vi "SetValue.vi"(8 "error in":errorcluster, 10 "Value":timestamp, 11 "DateTimeMeasure in":refnum<class "DateTimeMeasure.lvclass">) -> (0 "error out":errorcluster, 3 "DateTimeMeasure out":refnum<class "DateTimeMeasure.lvclass">)   [LabVIEW 2021, in "ProligentXMLGenerator.lvlib" / "DateTimeMeasure.lvclass"]
doc: "Defines the value acquired by the measure."
uses:
  DateTimeMeasure.lvclass
  DateTimeMeasure.lvclass/DateTimeMeasure.ctl
  Base/String_4000/String_4000.lvclass
  Base/DateTime/DateTime.lvclass
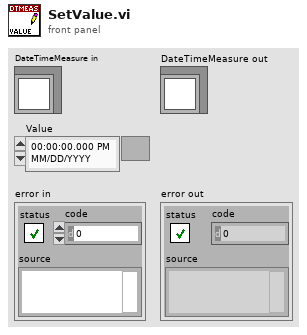
[diagram p1: front panel]
types:
  T1 = typedef "ProligentXMLGenerator.lvlib/DateTimeMeasure.lvclass/Data.ctl" = cluster{"Value":refnum<class "DateTime.lvclass">, "TimeZoneInfoId":string}
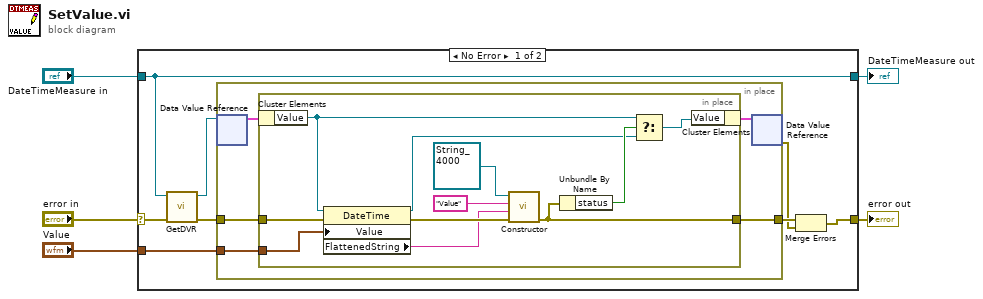
[diagram p0: block diagram]
diagram:
  n1 = case shown="No Error" "error in" {
    selector: "error in" -> [w9 w30]
    tunnel: "DateTimeMeasure in" -> [w10 w31]
    tunnel: [w12 w30] -> w3
    tunnel: "Value" -> [w11 _]
    tunnel: [w10 w31] -> w1
    frame No Error {
      n2 = call "GetDVR.vi"("error in"=w9, "DateTimeMeasure"=w10) -> ("error out"=w8:errorcluster, "DVRReference"=w13:refnum<data-value>)  [unwired: 8 in]
      n3 = in-place "In Place Element Structure" {
        in-place-border: w11 -> [w17]
        in-place-border: w8 -> [w18]
        in-place-border: [w16] -> w7
        n4 = in-place-dvr #1(w13) -> (w15:T1)  [unwired: 1 out]
        n5 = in-place "In Place Element Structure" {
          in-place-border: w18 -> [w29]
          in-place-border: w17 -> [w19]
          in-place-border: [w23] -> w16
          n6 = in-place-cluster #2(w15) -> ("Value"=w22:refnum<class "DateTime.lvclass">)
          n7 = property on="Property Node" class="DateTime"(reference=w22, error in=w29, "Value"=w19) -> (reference out=w21:refnum<class "DateTime.lvclass">, error out=w26:errorcluster, "FlattenedString"=w25:string)
          n8 = call-dynamic "Constructor.vi"("error in"=w26, "Value"=w25, "Name"="Value", "String in"=refnum<class "String_4000.lvclass"> refnum ("ProligentResultProcessor:String_4000")) -> ("error out"=w23:errorcluster)  [unwired: 6 in, 1 out]
          n9 = Unbundle By Name(w23) -> ("status"=w24:bool)
          n10 = Select(t=w22, s=w24, f=w21) -> (s? t:f=w20:refnum<class "DateTime.lvclass">)
          n11 = in-place-cluster #2("Value"=w20) -> (w14:T1)
        }
        n12 = in-place-dvr #1(w14) -> (w6:errorcluster)  [unwired: 1 out]
      }
      n13 = Merge Errors(w7, w6) -> (w12:errorcluster)
    }
    frame Error {
    }
  }
  "error out" <- w3
  "DateTimeMeasure out" <- w1
